vi "wait_file.vi"(7 "labHolo folder":string="..\\Images", 8 "error in (no error)":errorcluster, 9 "Wait min (s)":dbl=0.5 format="%#_13g", 10 "Timeout (s)":dbl=10.0 format="%#_13g", 11 "filename":string="beads_test_m+1_p0_a0_z4um.png") -> (0 "error out":errorcluster, 2 "done":bool)   [LabVIEW 2023]
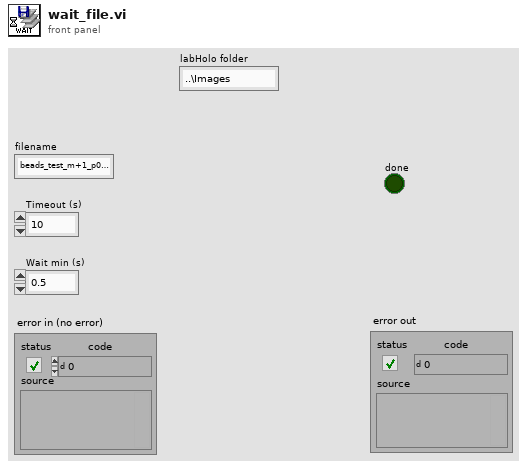
[diagram p1: front panel]
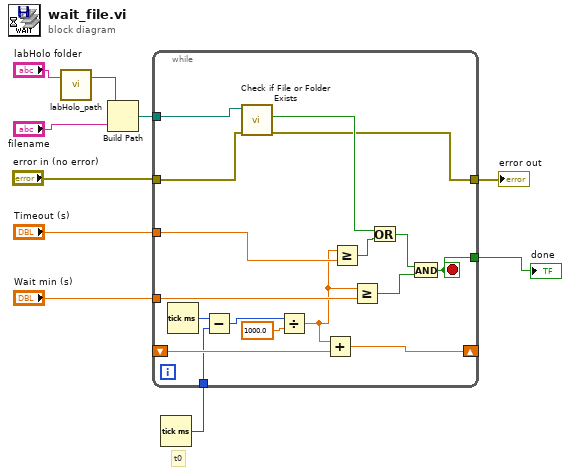
[diagram p0: block diagram]
diagram:
  # "t0"
  n1 = call "labHolo_path.vi"("sub folder or file (str)"="labHolo folder") -> ("labHolo path"=w3:path)  [unwired: 1 in, 1 out]
  n2 = Build Path(base path=w3, name or relative path="filename") -> (appended path=w2:path)
  n3 = Tick Count (ms)() -> (millisecond timer value=w5:u32)
  n4 = while {
    shift-right: [w26] -> _
    shift-left: _ -> [w27]
    tunnel: "Timeout (s)" -> [w24]
    tunnel: [w16] -> w8
    tunnel: "error in (no error)" -> [w17]
    tunnel: "Wait min (s)" -> [w19]
    tunnel: w5 -> [w14]
    tunnel: w2 -> [w12]
    tunnel: [w11] -> w1
    stop <- w11 stop-if-true
    n5 = Tick Count (ms)() -> (millisecond timer value=w15:u32)
    n6 = Subtract(x=w15, y=w14) -> (x-y=w13:u32)
    n7 = call <vilib>:"Check if File or Folder Exists.vi"("error in (no error)"=w17, "path"=w12) -> ("error out"=w16:errorcluster, "file or folder exists?"=w23:bool)  [unwired: 7 in, 1 out]
    n8 = Divide(x=w13, y=1000.0) -> (x/y=w18:dbl)
    n9 = Add(x=w18, y=w27) -> (x+y=w26:dbl)
    n10 = Greater Or Equal?(x=w18, y=w24) -> (x >= y?=w22:bool)
    n11 = Greater Or Equal?(x=w18, y=w19) -> (x >= y?=w21:bool)
    n12 = Or(x=w23, y=w22) -> (x .or. y?=w20:bool)
    n13 = And(x=w20, y=w21) -> (x .and. y?=w11:bool)
  }
  "error out" <- w8
  "done" <- w1
